vi "Get Object Parameter - 1D Array String.vi"(8 "error in (no error)":errorcluster, 9 "Default Value if JSON Null":string[](array[string]), 10 "Parameter Name":string, 11 "JSON Tree In (JSON Object)":variant) -> (0 "error out":errorcluster, 1 "is JSON Null?":bool, 2 "1D String Array Value":string[](array[string]), 3 "JSON Tree Out Passthrough":variant)   [LabVIEW 2011, in "i3-json.lvlib"]
doc: "Use this template to build a VI to use as a subVI."
uses:
  i3-json.lvlib
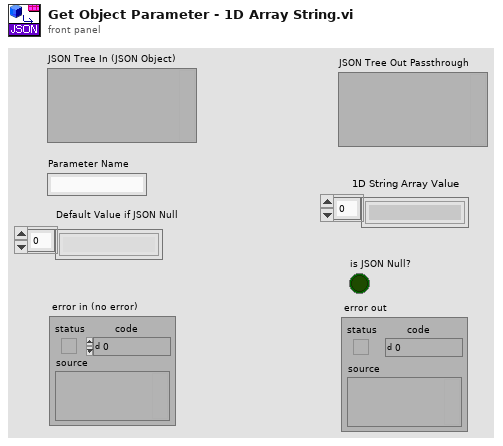
[diagram p1: front panel]
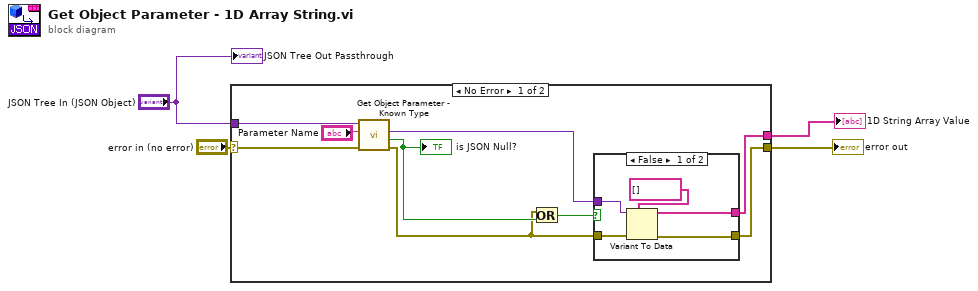
[diagram p0: block diagram]
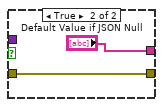
[diagram p2: hidden frame]
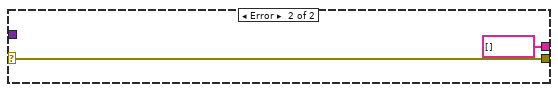
[diagram p3: hidden frame]
diagram:
  n1 = case shown="No Error" "error in (no error)" {
    selector: "error in (no error)" -> [w12 w22]
    tunnel: [w10 w22] -> w3
    tunnel: "JSON Tree In (JSON Object)" -> [w13 _]
    tunnel: [w7 string[] [] ("Default Value if JSON Null")] -> w2
    frame No Error {
      n2 = call "Get Object Parameter - Known Type.vi"("error in (no error)"=w12, "Parameter Name"="Parameter Name", "JSON Tree In (JSON Object)"=w13) -> ("error out"=w5:errorcluster, "is JSON Null?"=w8:bool, "Value"=w9:variant)  [unwired: 3 in, 3 out]
      "is JSON Null?" <- w8
      n3 = Or(x=w5, y=w8) -> (x .or. y?=w11:bool)
      n4 = case shown="False" w11 {
        tunnel: w5 -> [w18 w20]
        tunnel: [w15 w20] -> w10
        tunnel: w9 -> [w17 _]
        tunnel: [w16 "Default Value if JSON Null"] -> w7
        frame False {
          n5 = Variant To Data(error in=w18, type=string[] [], Variant=w17) -> (data=w16:string[], error out=w15:errorcluster)
        }
        frame True {
        }
      }
    }
    frame Error {
    }
  }
  "error out" <- w3
  "1D String Array Value" <- w2
  "JSON Tree Out Passthrough" <- "JSON Tree In (JSON Object)"
